vi "ECFEC Wrapper.vi"() -> (0 "error out":errorcluster)   [LabVIEW 2016, in "UT_Formatter.lvlib"]
uses:
  UT_Formatter.lvlib
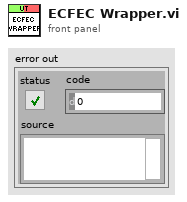
[diagram p1: front panel]
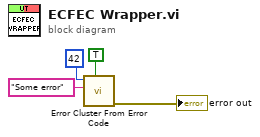
[diagram p0: block diagram]
diagram:
  n1 = call <vilib>:"Error Cluster From Error Code.vi"("show call chain? (False)"=TRUE, "error message (\"\")"="Some error" ("error message (\"\")"), "error code (0)"=42) -> ("error out"=→"error out":errorcluster)  [unwired: 6 in]
